vi "SubVI RX Rebuild Texts.vi"(8 "error in (no error)":errorcluster, 10 "input bit sequence":u8[](array[numeric])) -> (0 "error out":errorcluster, 2 "Received Message":string)   [LabVIEW 2015]
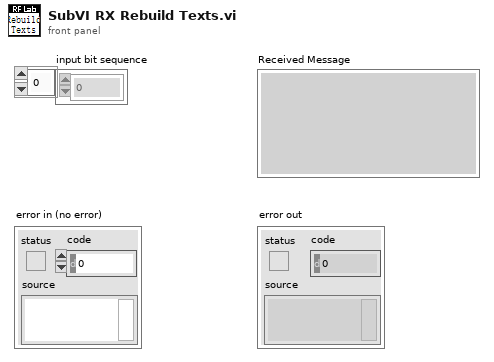
[diagram p1: front panel]
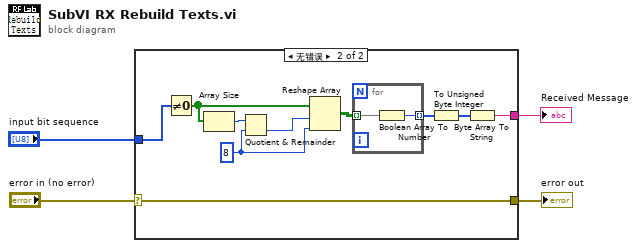
[diagram p0: block diagram]
diagram:
  n1 = case shown="无错误" "error in (no error)" {
    selector: "error in (no error)" -> [w5 w8]
    tunnel: [w5 w8] -> w3
    tunnel: "input bit sequence" -> [_ w7]
    tunnel: [_ w6] -> w1
    frame Error {
    }
    frame No Error {
      w12 = 8 ("dimension size")
      n2 = Not Equal To 0?(x=w7) -> (x != 0?=w14:bool[])
      n3 = Array Size(array=w14) -> (size(s)=w13:i32)
      n4 = Quotient & Remainder(x=w13, y=w12) -> (floor(x/y)=w15:i32)  [unwired: 1 out]
      n5 = Reshape Array(w14, w15, w12) -> (w11:bool[][])
      n6 = for {
        tunnel: w11 -> [w17] mode=indexing
        tunnel: [w16] -> w10 mode=indexing
        n7 = Boolean Array To Number(Boolean array=w17) -> (number=w16:u32)
      }
      n8 = To Unsigned Byte Integer(number=w10) -> (unsigned 8bit integer=w9:u8[])
      n9 = Byte Array To String(unsigned byte array=w9) -> (string=w6:string)
    }
  }
  "error out" <- w3
  "Received Message" <- w1
